vi "RT Loop - System Health and Monitoring.vi"(11 "Message Queue":refnum<queue>) -> ()   [LabVIEW 2022 SP3]
uses:
  support/Message Queue/Message Cluster.ctl
  controls/Control State.ctl
  Globals/Global - Configuration Options.vi
  <vilib>/nisyscfg/Close (System).vi
  <vilib>/NI_Real-Time Target Support.lvlib
  <vilib>/nisyscfg/nisyscfg.lvlib
  <resource>/objmgr/nisysapi.rc
  support/Message Queue/Message Queue.lvlib
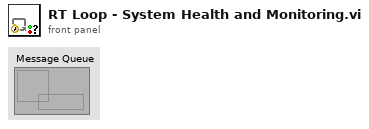
[diagram p1: front panel]
types:
  T1 = typedef "NI_Real-Time Target Support.lvlib/RT CPU Load.ctl" = cluster{"Total (%)":dbl, "Time Critical (%)":dbl, "Timed Structures (%)":dbl, "High (%)":dbl, "Above Normal (%)":dbl, "Normal (%)":dbl, "Background (%)":dbl, "Idle (%)":dbl, "ISR (%)":dbl}
  T2 = typedef "Control State.ctl" = enum16{"Safe State", "Manual", "Control (PID)"}
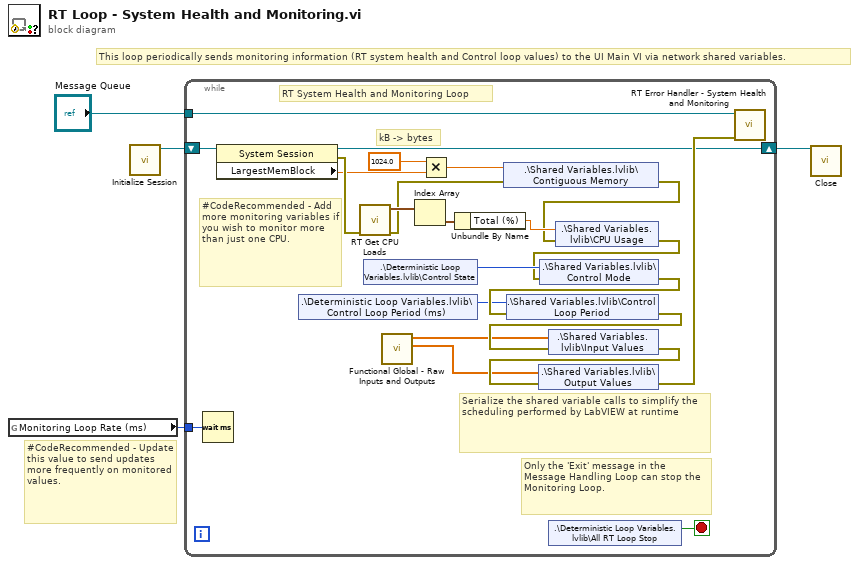
[diagram p0: block diagram]
diagram:
  # "#CodeRecommended - Update this value to send updates more frequently on monitored values."
  # "This loop periodically sends monitoring information (RT system health and Control loop values) to the UI Main VI via network shared variables."
  n1 = global read "Global - Configuration Options.vi" "Monitoring Loop Rate (ms)"() -> (w3:u32)
  n2 = call <vilib>:"Initialize Session.vi"() -> ("Session out"=w2:refnum<k21>)  [unwired: 10 in, 1 out]
  n3 = while {
    tunnel: "Message Queue" -> [w24]
    tunnel: w3 -> [w23]
    shift-right: [w9] -> w1
    shift-left: w2 -> [w13]
    stop <- w21 stop-if-true
    # "kB -> bytes"
    # "Serialize the shared variable calls to simplify the scheduling performed by LabVIEW at runtime"
    # "#CodeRecommended - Add more monitoring variables if you wish to monitor more than just one CPU."
    # "Only the 'Exit' message in the  Message Handling Loop can stop the Monitoring Loop."
    # "RT System Health and Monitoring Loop"
    n4 = Wait (ms)(milliseconds to wait=w23) -> ()  [unwired: 1 out]
    n5 = property class="System Session"(reference=w13) -> (reference out=w9:refnum<k21>, error out=w12:errorcluster, "LargestMemBlock"=w11:dbl)  [unwired: 1 in]
    n6 = shared-variable ".\\Deterministic Loop Variables.lvlib\\Control Loop Period (ms)"() -> (w19:u32)  [unwired: 1 in, 1 out]
    n7 = call <vilib>:"RT Get CPU Loads.vi"("error in (no error)"=w12) -> ("error out"=w10:errorcluster, "CPU loads"=w27:T1[])  [unwired: 9 in]
    n8 = shared-variable ".\\Deterministic Loop Variables.lvlib\\Control State"() -> (w20:T2)  [unwired: 1 in, 1 out]
    n9 = call "Functional Global - Raw Inputs and Outputs.vi"() -> ("Outputs out"=w14:dbl[], "Inputs out"=w15:dbl[])  [unwired: 10 in]
    n10 = Index Array(array=w27) -> (element=w26:T1)  [unwired: 1 in]
    n11 = Multiply(x=1024.0 ("y"), y=w11) -> (x*y=w5:dbl)
    n12 = Unbundle By Name(w26) -> ("Total (%)"=w25:dbl)
    n13 = shared-variable ".\\Shared Variables.lvlib\\Contiguous Memory"(w5, error in=w10) -> (error out=w8:errorcluster)
    n14 = shared-variable ".\\Deterministic Loop Variables.lvlib\\All RT Loop Stop"() -> (w21:bool)  [unwired: 1 in, 1 out]
    n15 = shared-variable ".\\Shared Variables.lvlib\\CPU Usage"(w25, error in=w8) -> (error out=w7:errorcluster)
    n16 = shared-variable ".\\Shared Variables.lvlib\\Control Mode"(w20, error in=w7) -> (error out=w22:errorcluster)
    n17 = shared-variable ".\\Shared Variables.lvlib\\Control Loop Period"(w19, error in=w22) -> (error out=w18:errorcluster)
    n18 = shared-variable ".\\Shared Variables.lvlib\\Input Values"(w15, error in=w18) -> (error out=w17:errorcluster)
    n19 = shared-variable ".\\Shared Variables.lvlib\\Output Values"(w14, error in=w17) -> (error out=w16:errorcluster)
    n20 = call "RT Error Handler - System Health and Monitoring.vi"("error in (no error)"=w16, "Message Queue"=w24) -> ()  [unwired: 9 in, 1 out]
  }
  n21 = call-poly <vilib>:"Close.vi"("Session in"=w1) -> ()  [unwired: 10 in, 1 out]
